vi "Test - Ignition.vi"(8 "error in":errorcluster, 10 "Boiler Configuration":T3, 11 "UI Data in":T1) -> (0 "error out":errorcluster, 3 "MHL Data":T1)   [LabVIEW 2014, in "Controller.lvlib"]
uses:
  Controller.lvlib
  controls/MHL UI Data.ctl
  controls/MHL Status.ctl
  Boiler/Boiler Configuration.ctl
  Boiler/Boiler.lvlib
  support/Message Queue/Message Queue.lvlib
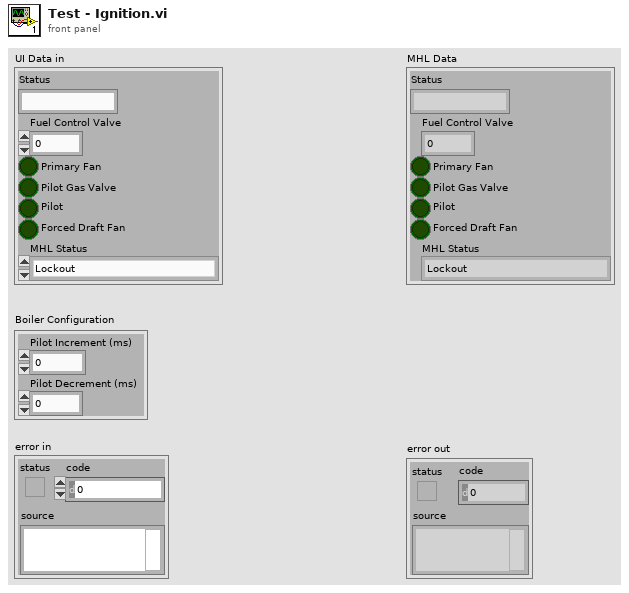
[diagram p1: front panel]
types:
  T1 = typedef "MHL UI Data.ctl" = cluster{"Status":string, "Fuel Control Valve":u32, "Primary Fan":bool, "Pilot Gas Valve":bool, "Pilot":bool, "Forced Draft Fan":bool, "MHL Status":T2}
  T2 = typedef "MHL Status.ctl" = enum16{"Lockout", "Ready", "Pre-Purge", "Pre-Purge Complete", "Pilot On", "Boiler Running", "Shutdown", "Purge"}
  T3 = typedef "Boiler.lvlib/Boiler Configuration.ctl" = cluster{"Pilot Increment (ms)":u32, "Pilot Decrement (ms)":u32}
  T4 = enum16{"open", "replace", "create", "open or create", "replace or create", "replace or create with confirmation"}
  T5 = typedef "Message Queue.lvlib/All Message Queues.ctl" = cluster{"MHL":refnum<queue>, "Boiler Controller":refnum<queue>, "Boiler":refnum<queue>}
  T6 = typedef "Notifiers.ctl" = cluster{"Handshake":refnum<notifier>, "Flame Level":refnum<notifier>, "Controller Exit":refnum<notifier>, "Boiler Exit":refnum<notifier>}
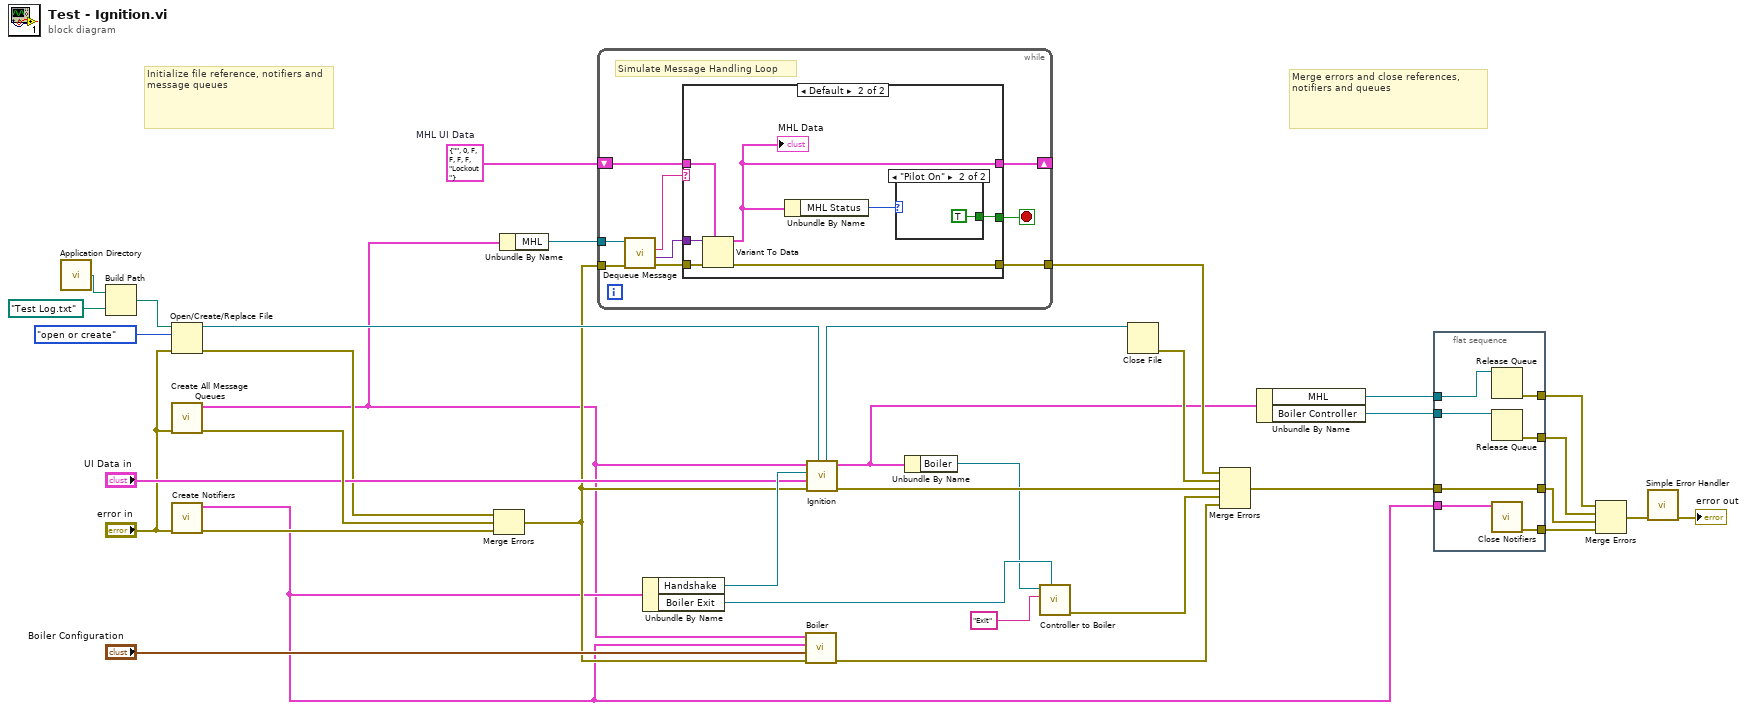
[diagram p0: block diagram]
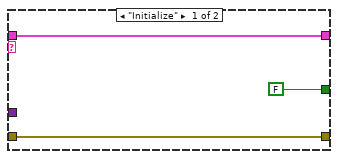
[diagram p2: hidden frame]
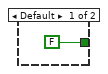
[diagram p3: hidden frame]
diagram:
  w21 = T1 {"Status"="", "Fuel Control Valve"=0, "Primary Fan"=FALSE, "Pilot Gas Valve"=FALSE, "Pilot"=FALSE, "Forced Draft Fan"=FALSE, "MHL Status"=enum."Lockout"}  # MHL UI Data
  # "Merge errors and close references, notifiers and queues"
  # "Initialize file reference, notifiers and message queues"
  n1 = call <vilib>:"Application Directory.vi"() -> ("Application Directory"=w32:path)
  n2 = Build Path(base path=w32, name or relative path=path "Test Log.txt") -> (appended path=w30:path)
  n3 = Open/Create/Replace File(file path (use dialog)=w30, error in="error in", operation (0:open)=T4."open or create") -> (refnum out=w27:refnum<file>, error out=w28:errorcluster)  [unwired: 3 in, 1 out]
  n4 = call "Create All Message Queues.vi"("error in"="error in") -> ("error out"=w34:errorcluster, "Message Queues out"=w5:T5)  [unwired: 9 in]
  n5 = call "Create Notifiers.vi"("error in"="error in") -> ("error out"=w35:errorcluster, "Notifiers"=w12:T6)  [unwired: 9 in]
  n6 = Merge Errors(w28, w34, w35) -> (w22:errorcluster)
  n7 = Unbundle By Name(w5) -> ("MHL"=w23:refnum<queue>)
  n8 = while {
    tunnel: w23 -> [w45]
    tunnel: w22 -> [w44]
    shift-right: [w41] -> _
    shift-left: w21 -> [w42]
    tunnel: [w38] -> w16
    stop <- w37 stop-if-true
    # "Simulate Message Handling Loop"
    n9 = call "Dequeue Message.vi"("error in (no error)"=w44, "Message Queue"=w45) -> ("error out"=w39:errorcluster, "Message Data"=w43:variant, "Message"=w40:string)  [unwired: 6 in, 1 out]
    n10 = case shown="Default" w40 {
      tunnel: w39 -> [w46 w55]
      tunnel: w43 -> [_ w54]
      tunnel: w42 -> [w48 w53]
      tunnel: [w48 w52] -> w41
      tunnel: [FALSE w50] -> w37
      tunnel: [w46 w49] -> w38
      frame "Initialize" {
      }
      frame Default {
        n11 = Variant To Data(error in=w55, type=w53, Variant=w54) -> (data=w52:T1, error out=w49:errorcluster)
        "MHL Data" <- w52
        n12 = Unbundle By Name(w52) -> ("MHL Status"=w51:T2)
        n13 = case shown="\"Pilot On\"" w51 {
          tunnel: [FALSE TRUE] -> w50
          frame Default {
          }
          frame "Pilot On" {
          }
        }
      }
    }
  }
  n14 = Unbundle By Name(w12) -> ("Handshake"=w36:refnum<notifier>, "Boiler Exit"=w9:refnum<notifier>)
  n15 = call "Boiler.vi"("error in"=w22, "Boiler Configuration"="Boiler Configuration", "Notifiers"=w12, "Message Queues"=w5) -> ("error out"=w2:errorcluster)  [unwired: 7 in]
  n16 = call "Ignition.vi"("Log File Refnum in"=w27, "error in"=w22, "UI Data in"="UI Data in", "Handshake Notifier in"=w36, "Message Queues in"=w5) -> ("error out"=w24:errorcluster, "Message Queues out"=w4:T5, "Log File Refnum out"=w18:refnum<file>)  [unwired: 2 in, 2 out]
  n17 = Unbundle By Name(w4) -> ("Boiler"=w3:refnum<queue>)
  n18 = call "Controller to Boiler.vi"("Notifier"=w9, "Message"="Exit", "Boiler Queue in"=w3) -> ("error out"=w1:errorcluster)  [unwired: 6 in, 2 out]
  n19 = Close File(refnum=w18) -> (error out=w17:errorcluster)  [unwired: 1 in, 1 out]
  n20 = Merge Errors(w16, w17, w24, w1, w2) -> (w6:errorcluster)
  n21 = Unbundle By Name(w4) -> ("MHL"=w19:refnum<queue>, "Boiler Controller"=w20:refnum<queue>)
  n22 = flat-sequence {
    tunnel: w20 -> [w64]
    tunnel: w19 -> [w63]
    tunnel: [w62] -> w14
    tunnel: [w61] -> w13
    tunnel: [w60] -> w8
    tunnel: w12 -> [w59]
    tunnel: [w58] -> w7
    tunnel: w6 -> [w58]
    frame #0 {
      n23 = Release Queue(queue=w63) -> (error out=w61:errorcluster)  [unwired: 2 in, 2 out]
      n24 = Release Queue(queue=w64) -> (error out=w62:errorcluster)  [unwired: 2 in, 2 out]
      n25 = call "Close Notifiers.vi"("Notifiers"=w59) -> ("error out"=w60:errorcluster)  [unwired: 10 in]
    }
  }
  n26 = Merge Errors(w13, w14, w7, w8) -> (w11:errorcluster)
  n27 = call <vilib>:"Simple Error Handler.vi"("error in (no error)"=w11) -> ("error out"=→"error out":errorcluster)  [unwired: 4 in, 4 out]
